vi "separate the given array in positive and negative array.vi"() -> ()   [LabVIEW 2012]
panel:
  out "Negative":dbl[](array[numeric])
  out "Positive":dbl[](array[numeric])
  in  "Array":dbl[](array[numeric])
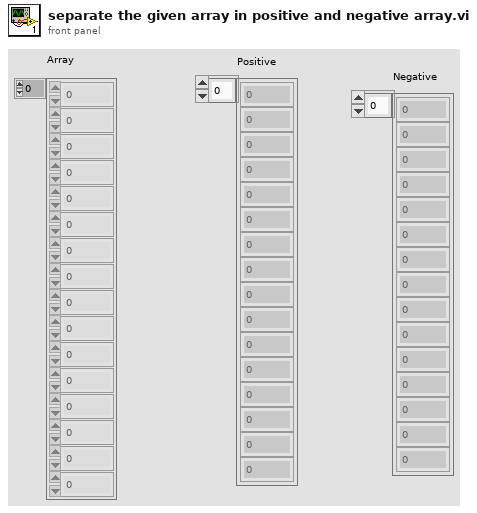
[diagram p1: front panel]
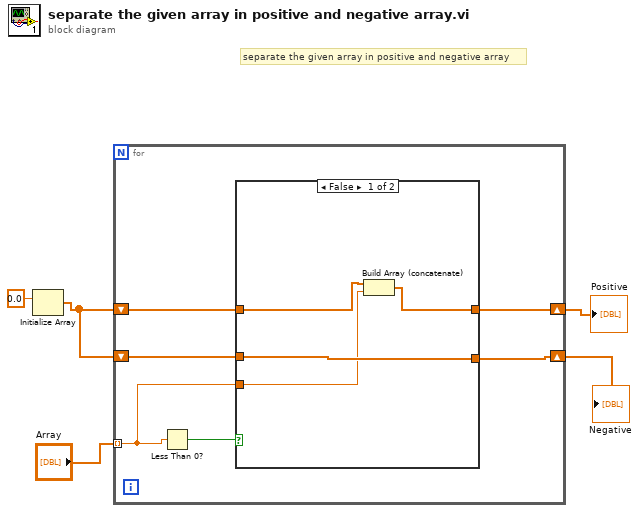
[diagram p0: block diagram]
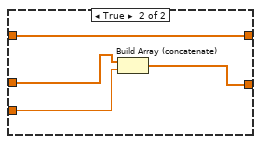
[diagram p2: hidden frame]
diagram:
  # "separate the given array in positive and negative array"
  n1 = Initialize Array(0.0 ("element")) -> (w4:dbl[])  [unwired: 1 in]
  n2 = for {
    shift-right: [w10] -> w2
    shift-left: w4 -> [w11]
    shift-right: [w9] -> w1
    shift-left: w4 -> [w8]
    tunnel: "Array" -> [w6] mode=indexing
    n3 = Less Than 0?(x=w6) -> (x < 0?=w7:bool)
    n4 = case shown="False" w7 {
      tunnel: w11 -> [w15 w19]
      tunnel: [w14 w19] -> w10
      tunnel: [w13 w17] -> w9
      tunnel: w8 -> [w13 w18]
      tunnel: w6 -> [w12 w16]
      frame False {
        n5 = Build Array (concatenate)(w15, w12) -> (w14:dbl[])
      }
      frame True {
        n6 = Build Array (concatenate)(w18, w16) -> (w17:dbl[])
      }
    }
  }
  "Positive" <- w2
  "Negative" <- w1
